vi "RequestStreaming RouteGuide Test.vi"() -> ()   [LabVIEW 2019, in "route_guide_client.lvlib"]
uses:
  route_guide_client.lvlib
  RPC Messages/routeguide_RouteSummary.ctl
panel:
  in  "error in":errorcluster
  out "error out":errorcluster
  in  "ms per iteration":u32=200
  in  "Longitude Loop":i32=4
  in  "Latitude Loop":i32=4
  out "Response Data":T1
  in  "Server Address":string="localhost:50051"
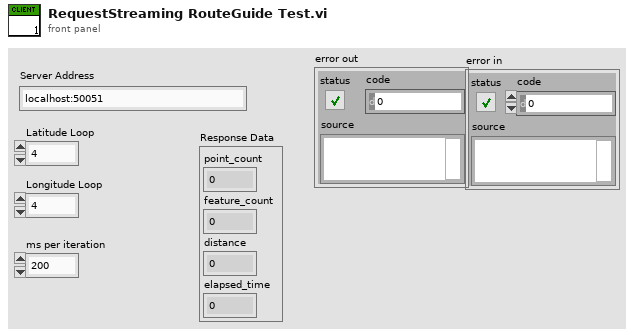
[diagram p1: front panel]
types:
  T1 = typedef "route_guide_client.lvlib/routeguide_RouteSummary.ctl" = cluster{"point_count":i32, "feature_count":i32, "distance":i32, "elapsed_time":i32}
  T2 = typedef "grpc-lvsupport-release.lvlib/grpcId.ctl" = u64
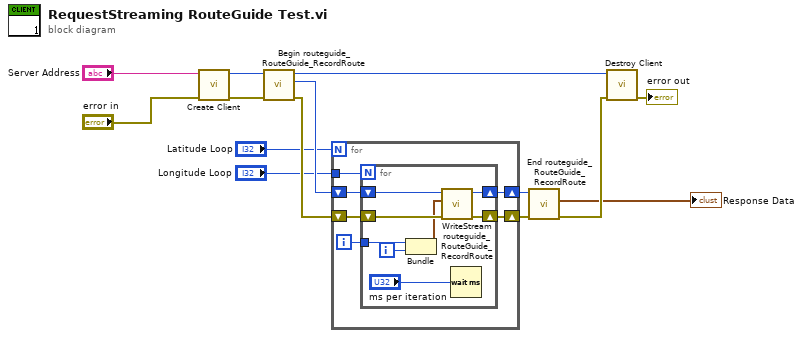
[diagram p0: block diagram]
diagram:
  n1 = call "Create Client.vi"("error in"="error in", "address"="Server Address") -> ("error out"=w12:errorcluster, "gRPC ID Out"=w13:T2)  [unwired: 8 in]
  n2 = call "Begin routeguide_RouteGuide_RecordRoute.vi"("error in"=w12, "gRPC ID"=w13) -> ("error out"=w10:errorcluster, "Call Id Out"=w11:T2, "gRPC ID out"=w6:T2)  [unwired: 7 in]
  n3 = for {
    N: "Latitude Loop" -> [_]
    shift-right: [w17] -> w8
    shift-left: w11 -> [w20]
    shift-right: [w18] -> w9
    shift-left: w10 -> [w19]
    tunnel: "Longitude Loop" -> [w15]
    i -> [w16]
    n4 = for {
      N: w15 -> [_]
      shift-right: [w25] -> w17
      shift-left: w20 -> [w28]
      shift-right: [w26] -> w18
      shift-left: w19 -> [w27]
      tunnel: w16 -> [w22]
      i -> [w24]
      n5 = Bundle(w22, w24) -> (w23:cluster{i32, i32})  [unwired: 1 in]
      n6 = call "WriteStream routeguide_RouteGuide_RecordRoute.vi"("error in"=w27, "Request Data"=w23, "Call ID in"=w28) -> ("error out"=w26:errorcluster, "Call ID"=w25:T2)  [unwired: 6 in, 1 out]
      n7 = Wait (ms)(milliseconds to wait="ms per iteration") -> ()  [unwired: 1 out]
    }
  }
  n8 = call "End routeguide_RouteGuide_RecordRoute.vi"("error in"=w9, "Call ID in"=w8) -> ("error out"=w7:errorcluster, "Response Data"=→"Response Data":T1)  [unwired: 7 in, 1 out]
  n9 = call "Destroy Client.vi"("error in"=w7, "gRPC ID"=w6) -> ("error out"=→"error out":errorcluster)  [unwired: 9 in]
